vi "Control Panel No Objects.vi"(8 "error in (no error)":errorcluster) -> (0 "error out":errorcluster)   [LabVIEW 2009]
doc: "(Dynamic) A user-level application that simulates the physical front panel of the Instrument. Provide the user with buttons to manually control features of the instrument, and provide indicators of its current state."
uses:
  Math Operations/To Start and Stop (bare).vi
  Math Operations/To Center and Span (frequency).vi
  Function Generator.lvclass
  Tektronix AFG 3000 Series/Tektronix AFG 3000 Series.lvlib
  Tektronix AFG 3000 Series/controls.llb/Channel.ctl
  Math Operations/To Center and Span (bare).vi
  Math Operations/To Start and Stop (frequency).vi
  Tektronix AFG 3000 Series/controls.llb/Voltage.ctl
  Tektronix AFG 3000 Series/controls.llb/Frequency Mode.ctl
  Tektronix AFG 3000 Series/controls.llb/Sweep Frequency.ctl
  Tektronix AFG 3000 Series/controls.llb/Sweep Time Parameter.ctl
  Global/GPIB Numbers.vi
  Tektronix AFG 3000 Series/controls.llb/Waveform Shape.ctl
  Tektronix AFG 3000 Series/controls.llb/Sweep Spacing.ctl
panel:
  in  "Initial Cluster":T1
  in  "Ch2 on/off":bool
  in  "Ch1 on/off":bool
  out "Ready when blinking":bool
  in  "Set":bool
  in  "Read to control":bool
  in  "Read":bool
  in  "Copy actual to set":bool
  in  "Populate fields with member data":bool
  out "Start Freq.":dbl[unit]
  out "Stop Freq.":dbl[unit]
  out "Freq. Span":dbl[unit]
  out "Center Freq.":dbl[unit]
  out "Offset":dbl[unit]
  out "Amplitude":dbl[unit]
  out "High":dbl[unit]
  out "Low":dbl[unit]
  out "FM Source":u16(ring) items=["Internal", "External"]
  out "FM Modulation Waveform":u16(ring) items=["Sine", "Square", "Triangle", "Ramp", "Down Ramp", "Noise", "User 1", "User 2", "User 3", "User 4", "EMEMory", "EFILe"]
  out "FM Modulation Freq.":dbl[unit]=100.0
  out "FM Peak Deviation":dbl[unit]=100.0
  in  "FM Peak Deviation Set":dbl[unit]=100.0
  in  "FM Modulation Freq Set":dbl[unit]=100.0
  in  "FM Modulation Waveform Set":u16(ring) items=["Sine", "Square", "Triangle", "Ramp", "Down Ramp", "Noise", "User 1", "User 2", "User 3", "User 4", "EMEMory", "EFILe"]
  in  "FM Source Set":u16(ring) items=["Internal", "External"]
  out "AM Modulation Freq.":dbl[unit]=1000.0
  out "AM Modulation Waveform":u16(ring) items=["Sine", "Square", "Triangle", "Ramp", "Down Ramp", "Noise"]
  out "AM Source":u16(ring) items=["Internal", "External"]
  out "AM Modulation Depth":dbl
  in  "AM Modulation Depth Set":dbl
  in  "AM Modulation Freq. Set":dbl[unit]=1000.0
  in  "AM Modulation Waveform Set":u16(ring) items=["Sine", "Square", "Triangle", "Ramp", "Down Ramp", "Noise"]
  in  "AM Source Set":u16(ring) items=["Internal", "External"]
  out "Return Time":dbl[unit]
  out "Hold Time":dbl[unit]
  out "Sweep Time":dbl[unit]
  in  "Return Time Set":dbl[unit]
  in  "Hold Time Set":dbl[unit]
  in  "Sweep Time Set":dbl[unit] caption="Sweep time"
  out "Sweep Spacing":T2 items=["linear", "log"]
  in  "Sweep Spacing Set":T2 items=["linear", "log"]
  in  "Stop Freq. Set":dbl[unit]
  in  "Start Freq. Set":dbl[unit]
  out "Burst Mode":u16(ring)=1 items=["Triggered", "Gated"]
  out "Burst Count":i32=5
  in  "Burst Count Set":i32=5
  in  "Burst Mode Set":u16(ring)=1 items=["Triggered", "Gated"]
  out "Run Mode":u16(ring) items=["Continuous", "AM", "FM", "PM", "FSK", "PWM", "Sweep", "Burst"]
  in  "Run Mode Set":u16(ring) items=["Continuous", "AM", "FM", "PM", "FSK", "PWM", "Sweep", "Burst"]
  out "Trailing Edge Time":dbl[unit]
  out "Leading Edge Time":dbl[unit]
  out "Duty Cycle (%)":dbl
  in  "Duty Cycle Set (%)":dbl=50.0
  in  "Trailing Edge Time Set":dbl[unit]=5e-09 format="%#.6g"
  in  "Leading Edge Time Set":dbl[unit]=5e-09 format="%#.6g"
  out "Ramp Symm. (%)":dbl
  in  "Ramp Symm. Set (%)":dbl=50.0 min=0.0 max=100.0 step=1.0 format="%.2f"
  in  "Freq. Span Set":dbl[unit]
  in  "Center Freq. Set":dbl[unit]
  in  "Low Set":dbl[unit]
  in  "High Set":dbl[unit]
  in  "Amplitude Set":dbl[unit]
  in  "Offset Set":dbl[unit]
  in  "Exit":bool
  out "Waveform Shape":T3 items=["Sinusoid", "Square", "Pulse", "Ramp", "PRNoise", "DC", "SINC", "Gaussian", "Lorentz", "ERise", "EDecay", "Haversine", "User 1", "User 2", "User 3", "User 4", "EMemory", "EFile"]
  in  "Waveform Shape Set":T3 items=["Sinusoid", "Square", "Pulse", "Ramp", "PRNoise", "DC", "SINC", "Gaussian", "Lorentz", "ERise", "EDecay", "Haversine", "User 1", "User 2", "User 3", "User 4", "EMemory", "EFile"]
  out "Phase":dbl[unit]
  in  "Phase Set":dbl[unit]
  out "Frequency":dbl[unit]
  in  "Frequency Set":dbl[unit]
  in  "Channel":T4 items=["Channel 1", "Channel 2"]
  # "Tektronix AFG252 Function Generator Control Panel"
  # "VOLTAGE SETTINGS"
  # "SWEEP MODE SETTINGS"
  # "AM SETTINGS"
  # "GENERAL SETTINGS"
  # "RAMP SETTINGS"
  # "FM SETTINGS"
  # "Note: the program only sets\nthe values that are appropriate\nfor the run mode you select. I.e.,\nit won't set the FM settings if you\nselect \"Burst Mode\" here."
  # "PULSE SETTINGS"
  # "BURST MODE SETTINGS"
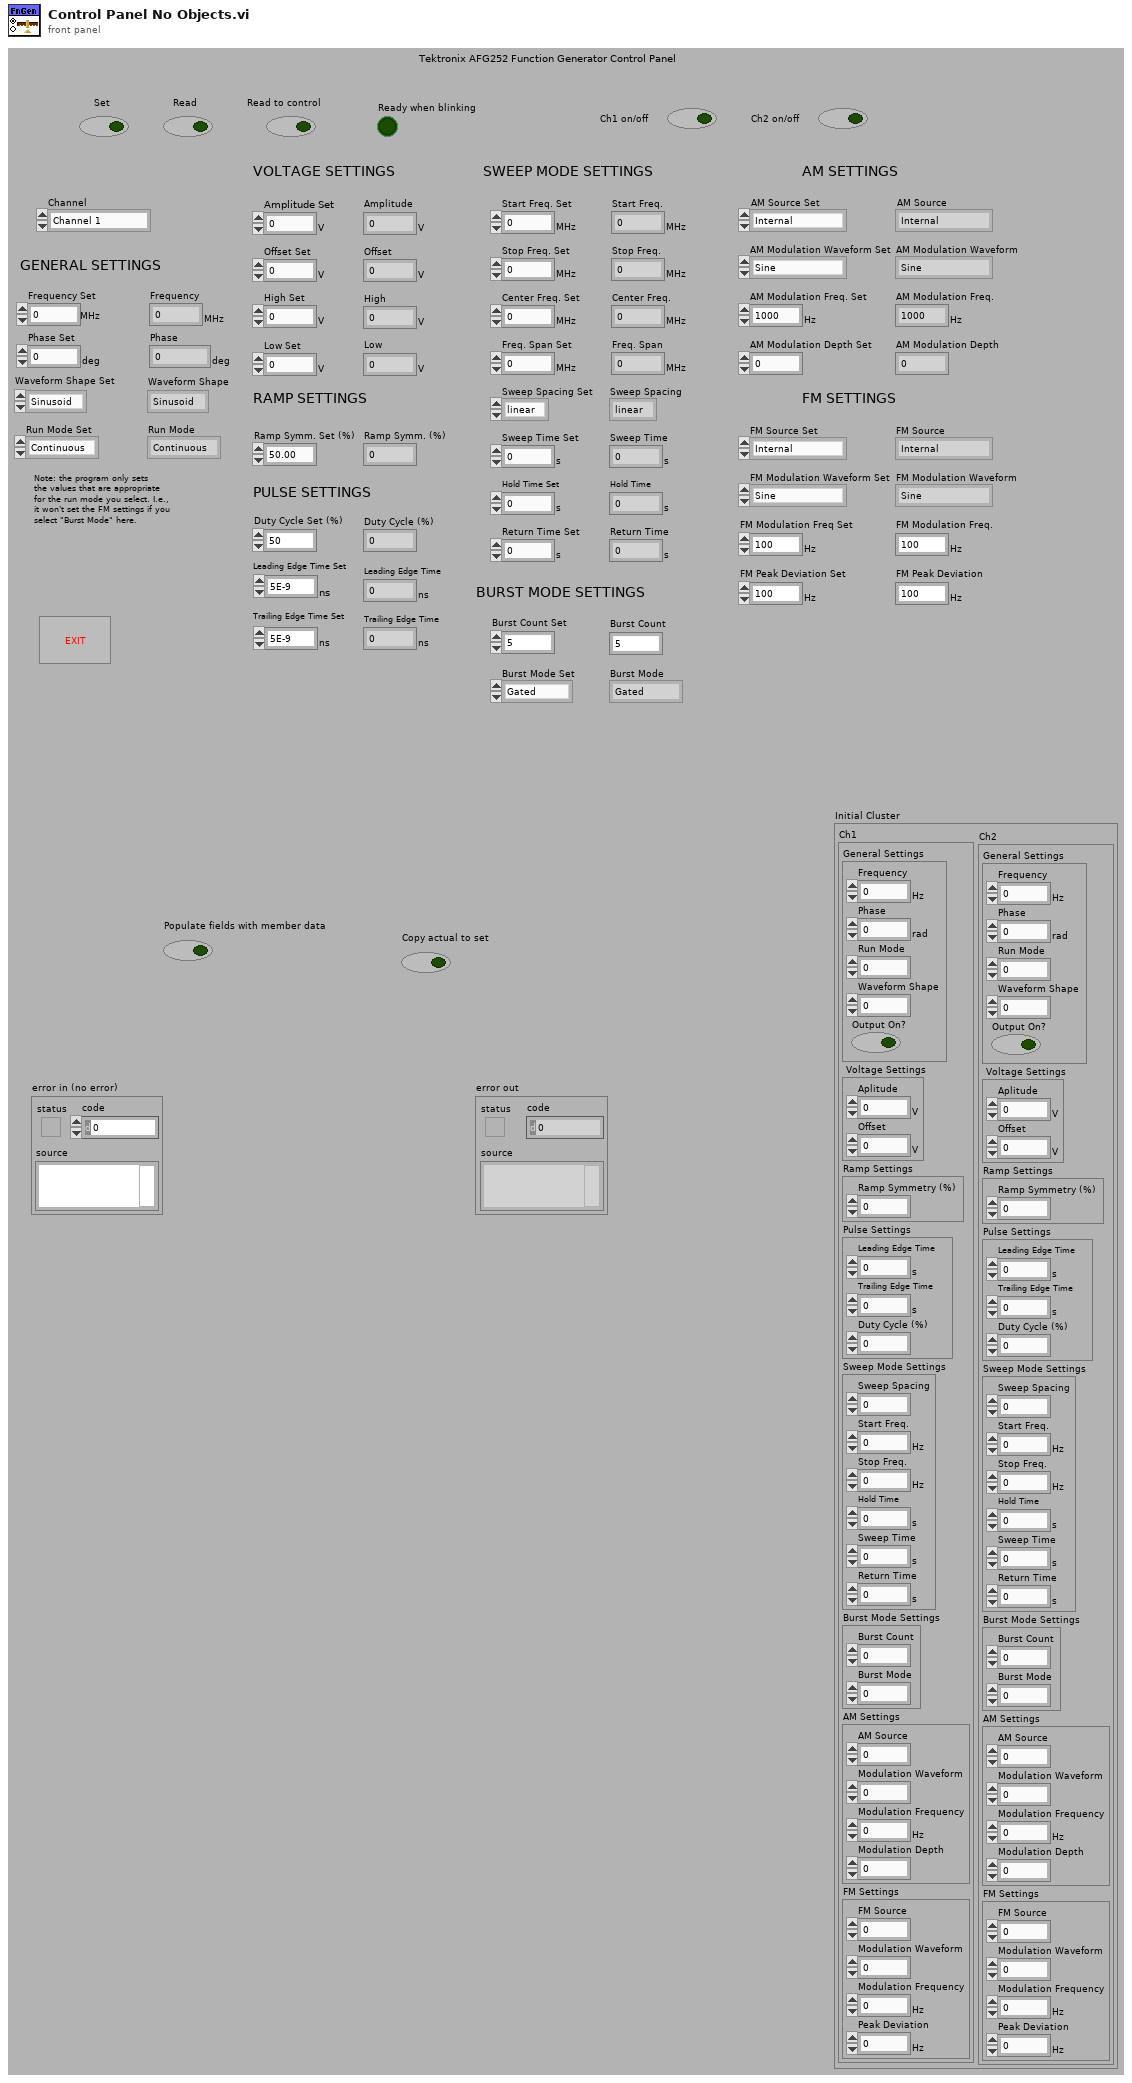
[diagram p1: front panel]
types:
  T1 = cluster{"Ch1":cluster{"General Settings":cluster{"Frequency":dbl[unit], "Phase":dbl[unit], "Run Mode":u16, "Waveform Shape":u16, "Output On?":bool}, " Voltage Settings":cluster{"Aplitude":dbl[unit], "Offset":dbl[unit]}, "Ramp Settings":cluster{"Ramp Symmetry (%)":dbl}, "Pulse Settings":cluster{"Leading Edge Time":dbl[unit], "Trailing Edge Time":dbl[unit], "Duty Cycle (%)":dbl}, "Sweep Mode Settings":cluster{"Sweep Spacing":u16, "Start Freq.":dbl[unit], "Stop Freq.":dbl[unit], "Hold Time":dbl[unit], "Sweep Time":dbl[unit], "Return Time":dbl[unit]}, "Burst Mode Settings":cluster{"Burst Count":i32, "Burst Mode":u16}, "AM Settings":cluster{"AM Source":u16, "Modulation Waveform":u16, "Modulation Frequency":dbl[unit], "Modulation Depth":dbl}, "FM Settings":cluster{"FM Source":u16, "Modulation Waveform":u16, "Modulation Frequency":dbl[unit], "Peak Deviation":dbl[unit]}}, "Ch2":cluster{"General Settings":cluster{"Frequency":dbl[unit], "Phase":dbl[unit], "Run Mode":u16, "Waveform Shape":u16, "Output On?":bool}, " Voltage Settings":cluster{"Aplitude":dbl[unit], "Offset":dbl[unit]}, "Ramp Settings":cluster{"Ramp Symmetry (%)":dbl}, "Pulse Settings":cluster{"Leading Edge Time":dbl[unit], "Trailing Edge Time":dbl[unit], "Duty Cycle (%)":dbl}, "Sweep Mode Settings":cluster{"Sweep Spacing":u16, "Start Freq.":dbl[unit], "Stop Freq.":dbl[unit], "Hold Time":dbl[unit], "Sweep Time":dbl[unit], "Return Time":dbl[unit]}, "Burst Mode Settings":cluster{"Burst Count":i32, "Burst Mode":u16}, "AM Settings":cluster{"AM Source":u16, "Modulation Waveform":u16, "Modulation Frequency":dbl[unit], "Modulation Depth":dbl}, "FM Settings":cluster{"FM Source":u16, "Modulation Waveform":u16, "Modulation Frequency":dbl[unit], "Peak Deviation":dbl[unit]}}}
  T2 = typedef "Sweep Spacing.ctl" = u16
  T3 = typedef "Waveform Shape.ctl" = u16
  T4 = typedef "Channel.ctl" = u16
  T5 = typedef "Voltage.ctl" = enum16{"amplitude", "offset", "high", "low", "high limit", "low limit"}
  T6 = typedef "Frequency Mode.ctl" = enum16{"CW", "Sweep"}
  T7 = typedef "Sweep Time Parameter.ctl" = enum16{"sweep time", "hold time", "return time"}
  T8 = typedef "Sweep Frequency.ctl" = enum16{"center", "span", "start", "stop"}
  T9 = cluster{"General Settings":cluster{"Frequency":dbl[unit], "Phase":dbl[unit], "Run Mode":u16, "Waveform Shape":u16, "Output On?":bool}, " Voltage Settings":cluster{"Aplitude":dbl[unit], "Offset":dbl[unit]}, "Ramp Settings":cluster{"Ramp Symmetry (%)":dbl}, "Pulse Settings":cluster{"Leading Edge Time":dbl[unit], "Trailing Edge Time":dbl[unit], "Duty Cycle (%)":dbl}, "Sweep Mode Settings":cluster{"Sweep Spacing":u16, "Start Freq.":dbl[unit], "Stop Freq.":dbl[unit], "Hold Time":dbl[unit], "Sweep Time":dbl[unit], "Return Time":dbl[unit]}, "Burst Mode Settings":cluster{"Burst Count":i32, "Burst Mode":u16}, "AM Settings":cluster{"AM Source":u16, "Modulation Waveform":u16, "Modulation Frequency":dbl[unit], "Modulation Depth":dbl}, "FM Settings":cluster{"FM Source":u16, "Modulation Waveform":u16, "Modulation Frequency":dbl[unit], "Peak Deviation":dbl[unit]}}
  T10 = cluster{"General Settings":cluster{"Frequency":dbl[unit], "Phase":dbl[unit], "Run Mode":u16, "Waveform Shape":u16, "Output On?":bool}, " Voltage Settings":cluster{"Aplitude":dbl[unit], "Offset":dbl[unit]}, "Ramp Settings":cluster{"Ramp Symmetry (%)":dbl}, "Pulse Settings":cluster{"Leading Edge Time":dbl[unit], "Trailing Edge Time":dbl[unit], "Duty Cycle (%)":dbl}, "Sweep Mode Settings":cluster{"Sweep Spacing":u16, "Start Freq.":dbl[unit], "Stop Freq.":dbl[unit], "Hold Time":dbl[unit], "Sweep Time":dbl[unit], "Return Time":dbl[unit]}, "Burst Mode Settings":cluster{"Burst Count":i32, "Burst Mode":u16}, "AM Settings":cluster{"AM Source":u16, "Modulation Waveform":u16, "Modulation Frequency":dbl[unit], "Modulation Depth":dbl}, "FM Settings":cluster{"FM Source":u16, "Modulation Waveform":u16, "Modulation Frequency":dbl[unit], "Peak Deviation":dbl[unit]}}[]
  T11 = typedef "GPIB Type Def.ctl" = cluster{"Name":string, "bus":dbl, "GPIB":dbl, "GPIB as string":string, "byte":i32, "VISA Resource Name":refnum<visa-resource-name>}
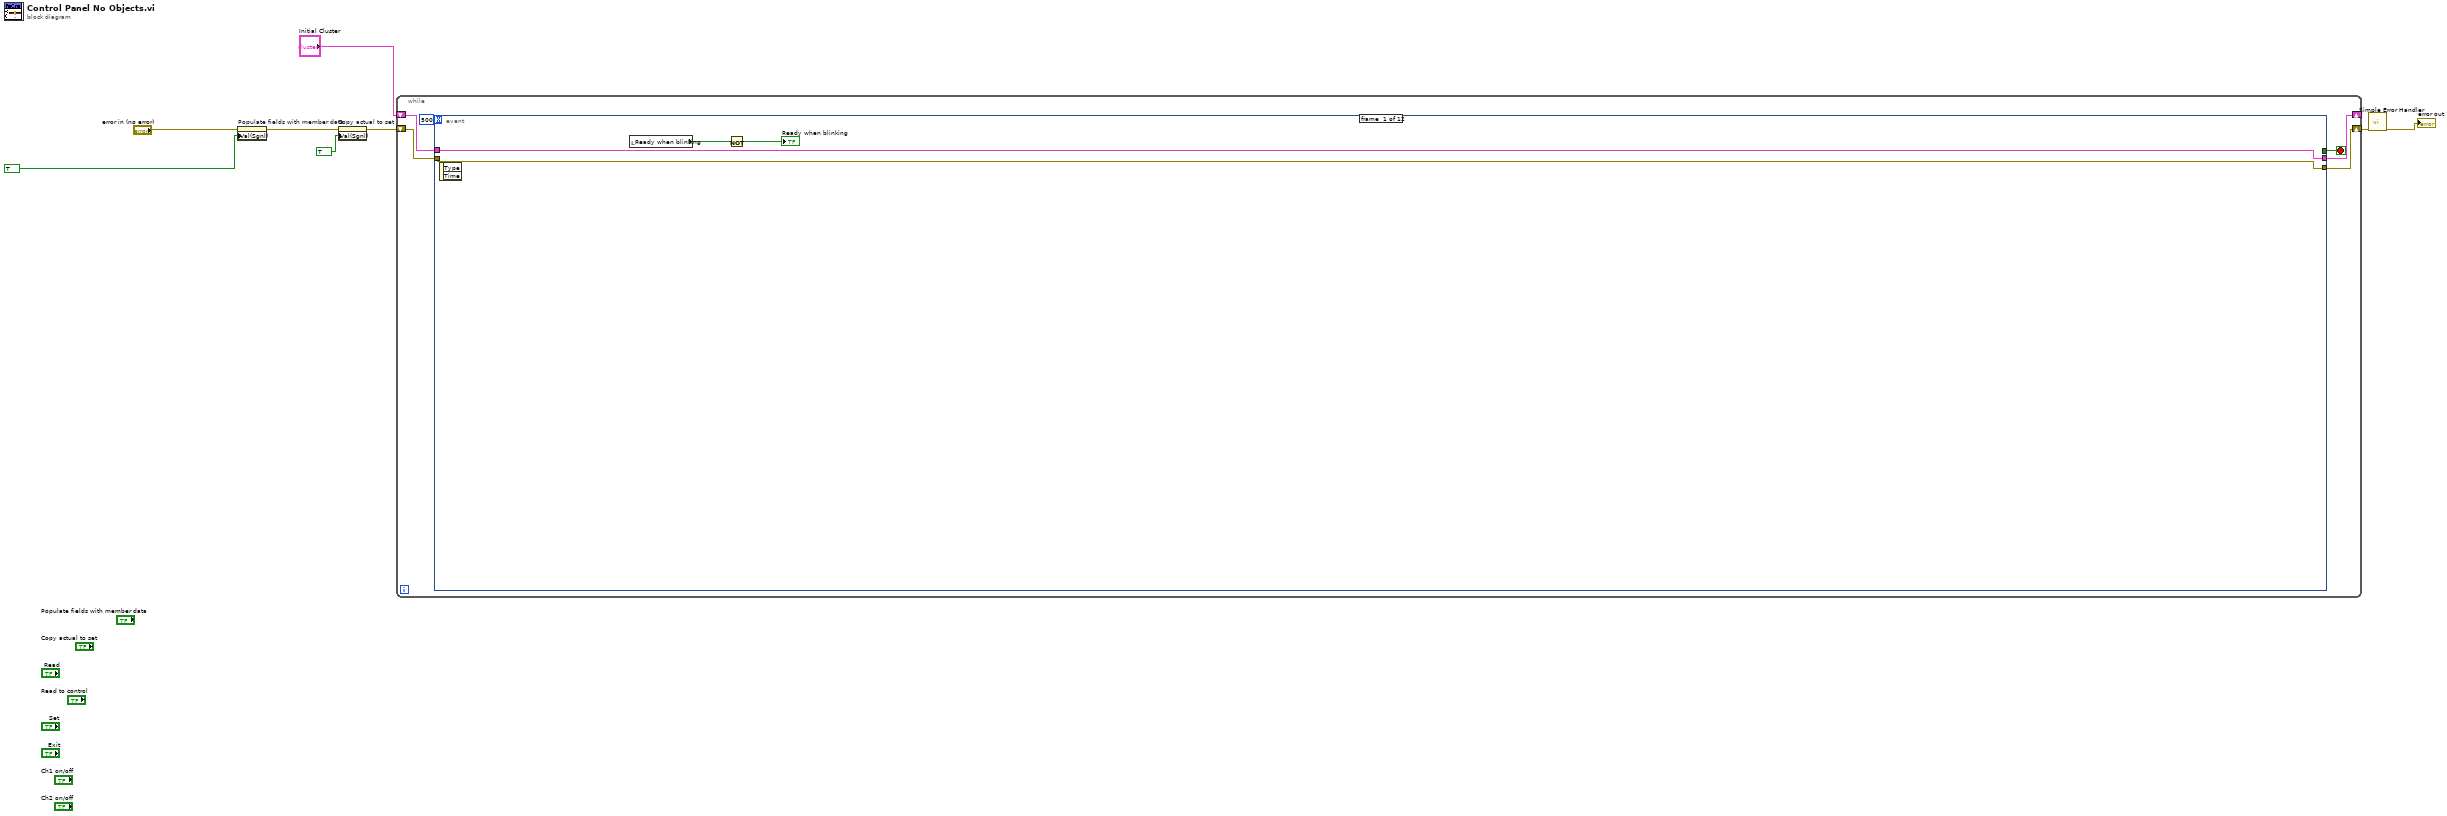
[diagram p0: block diagram]
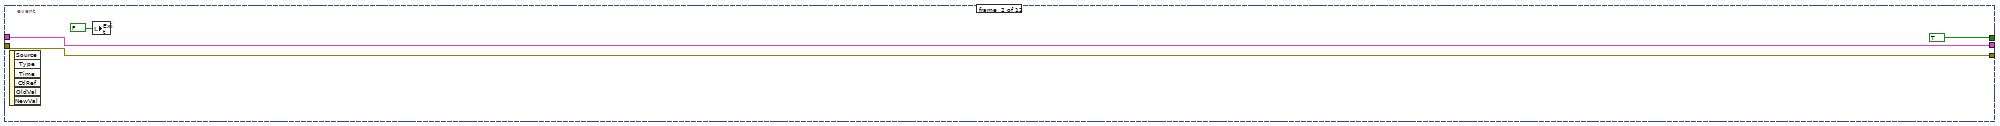
[diagram p2: hidden frame]
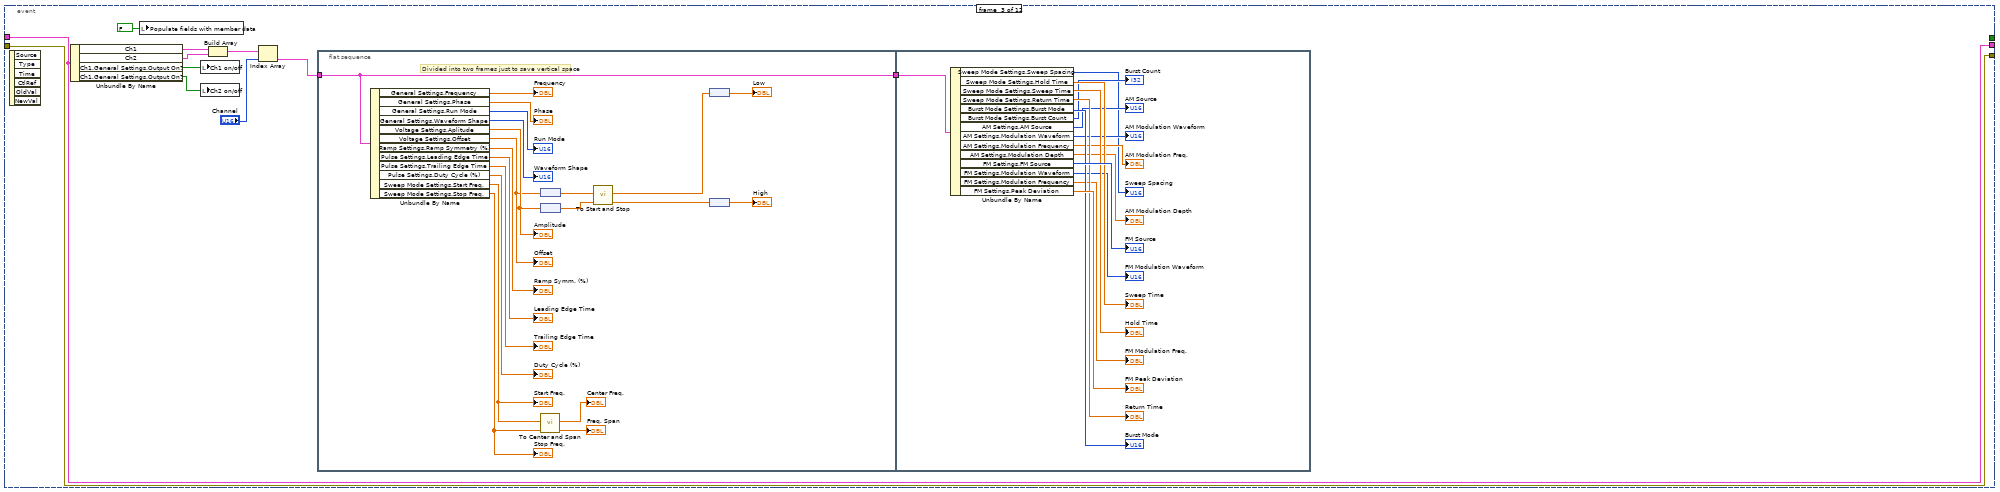
[diagram p3: hidden frame]
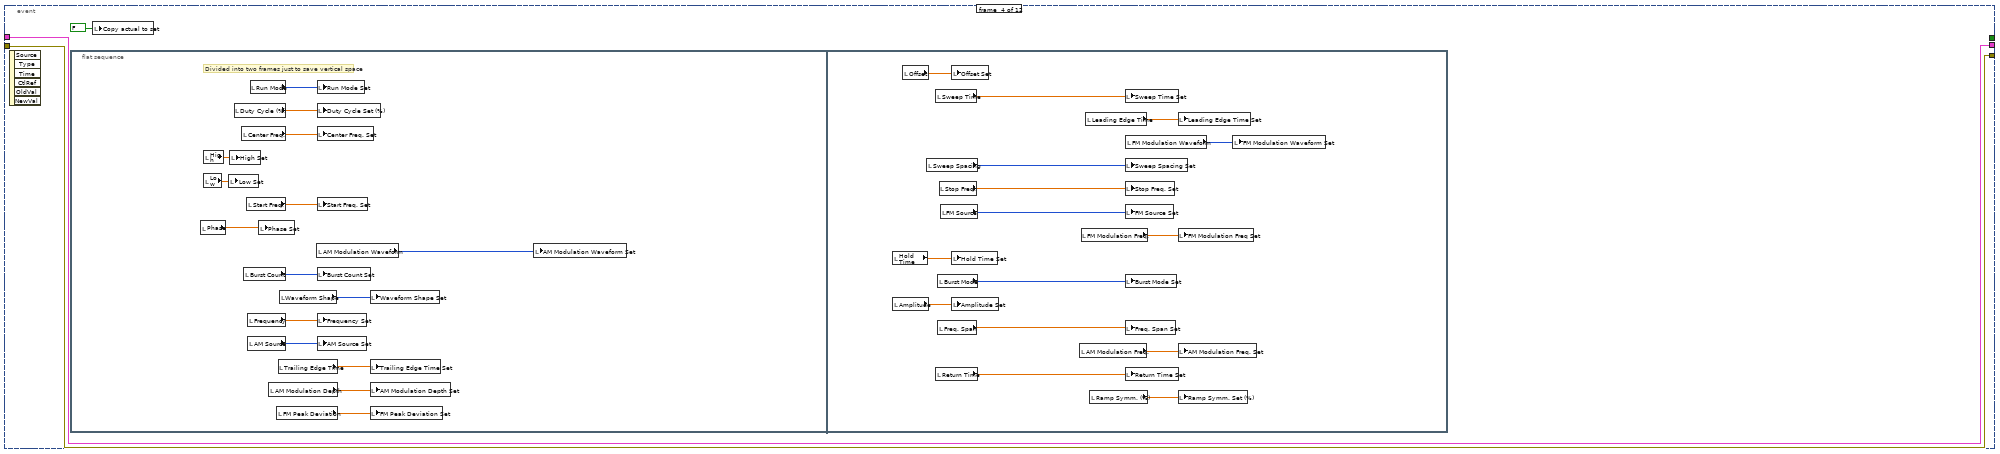
[diagram p4: hidden frame]
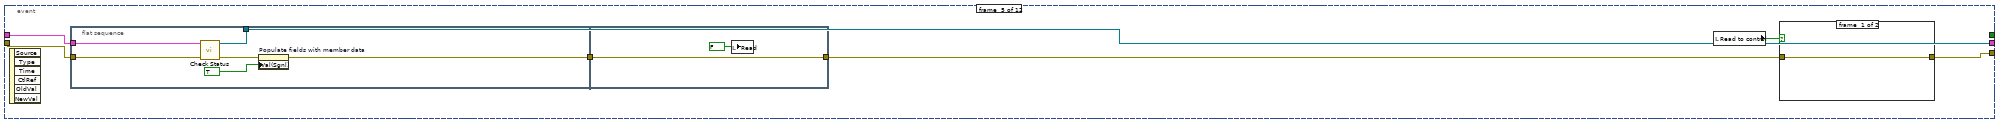
[diagram p5: hidden frame]
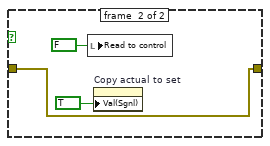
[diagram p6: hidden frame]
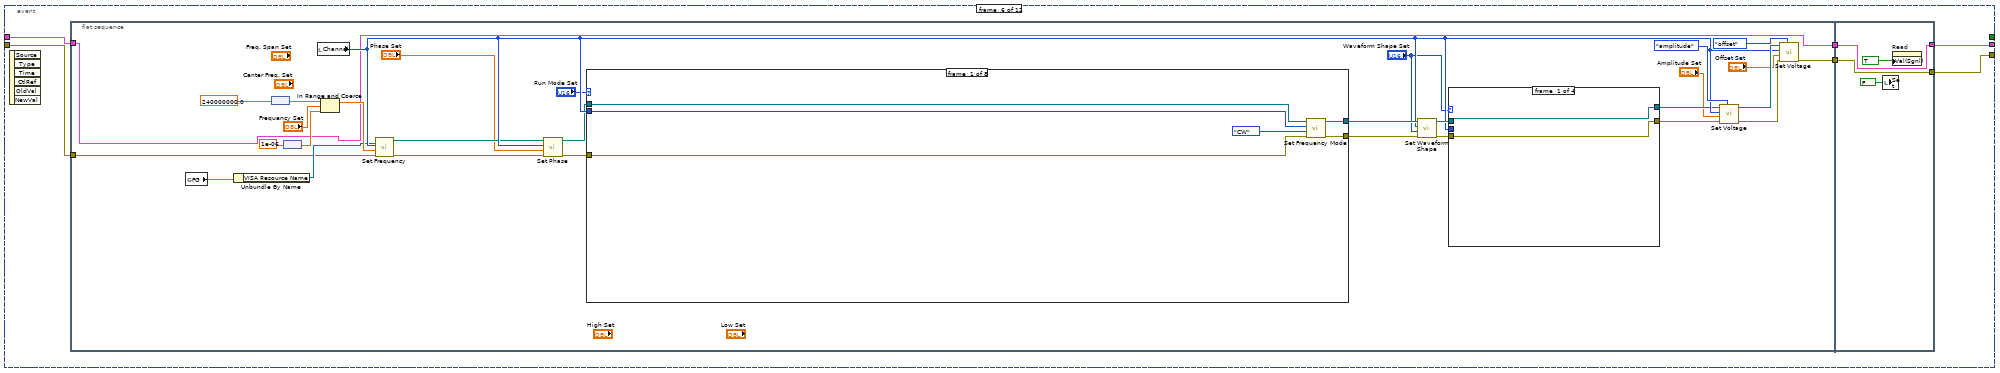
[diagram p7: hidden frame]
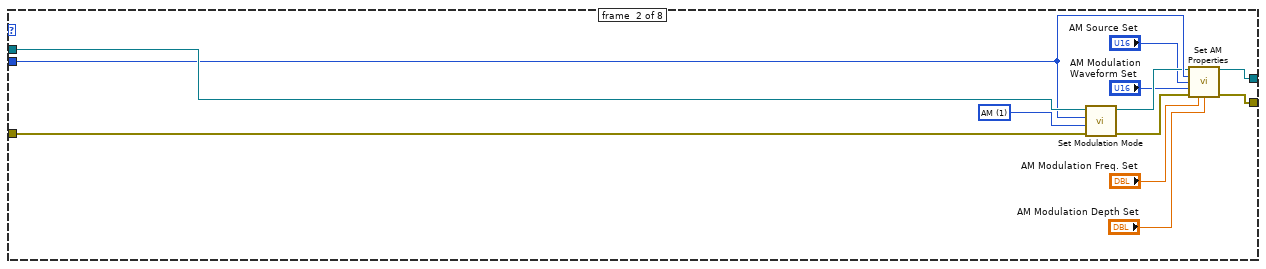
[diagram p8: hidden frame]
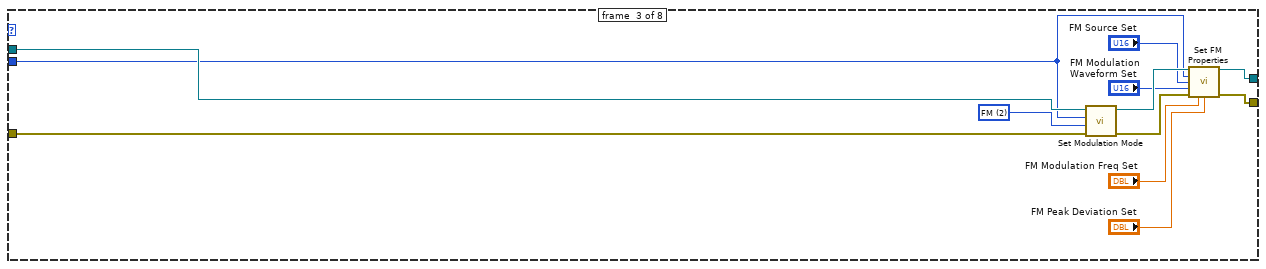
[diagram p9: hidden frame]
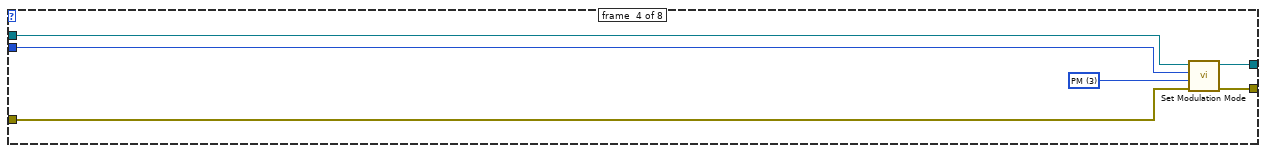
[diagram p10: hidden frame]
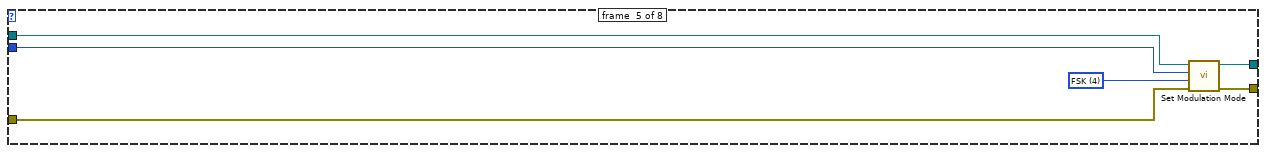
[diagram p11: hidden frame]
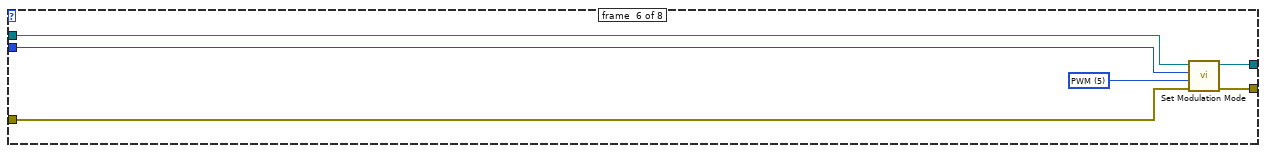
[diagram p12: hidden frame]
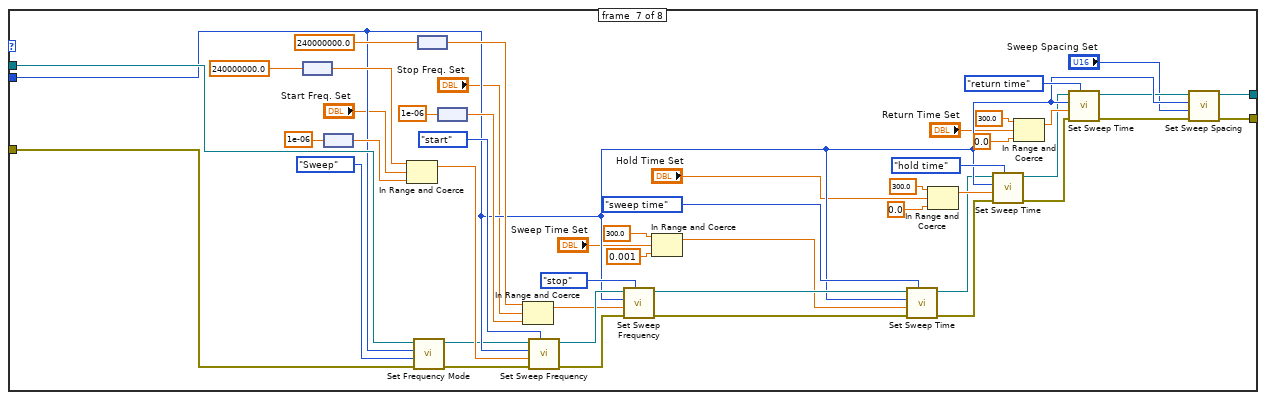
[diagram p13: hidden frame]
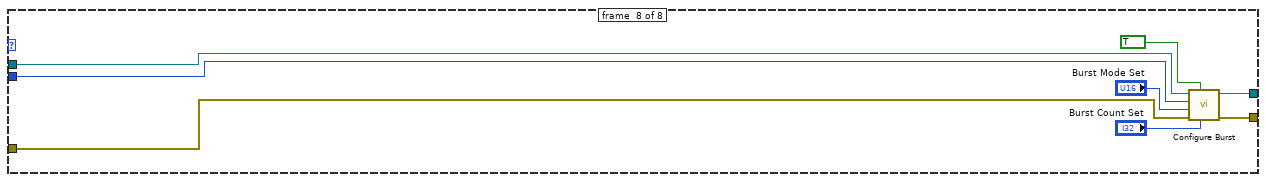
[diagram p14: hidden frame]
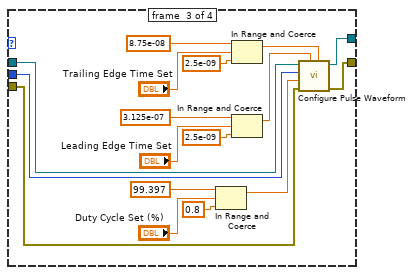
[diagram p16: hidden frame]
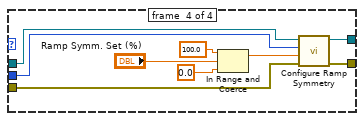
[diagram p17: hidden frame]
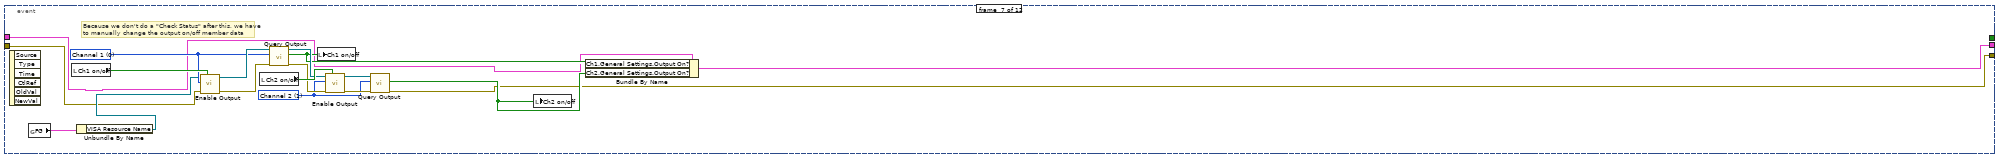
[diagram p18: hidden frame]
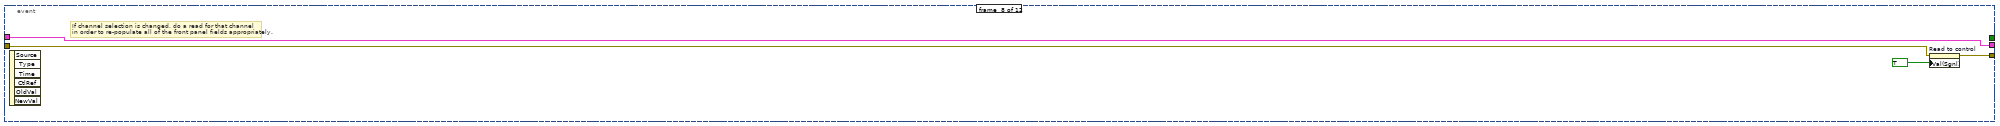
[diagram p19: hidden frame]
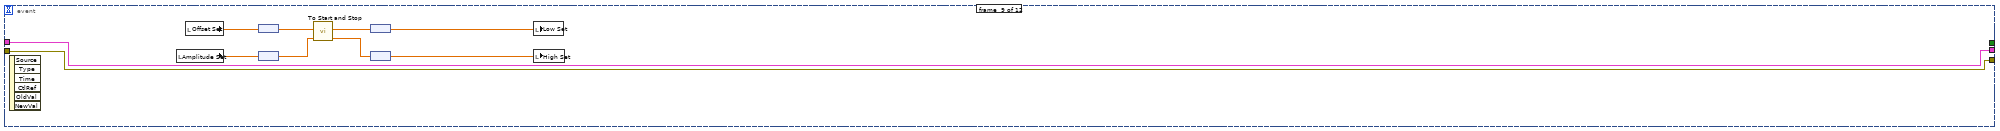
[diagram p20: hidden frame]
diagram:
  n1 = property on="Populate fields with member data" class="Bool (strict)"(error in="error in (no error)", "Val(Sgnl)"=TRUE ("Value (Signaling)")) -> (error out=w6:errorcluster)  [unwired: 1 in, 1 out]
  n2 = property on="Copy actual to set" class="Bool (strict)"(error in=w6, "Val(Sgnl)"=TRUE ("Value (Signaling)")) -> (error out=w5:errorcluster)  [unwired: 1 in, 1 out]
  n3 = while {
    shift-right: [w14] -> w4
    shift-left: w5 -> [w13]
    shift-right: [w11] -> _
    shift-left: "Initial Cluster" -> [w12]
    stop <- w9 stop-if-true
    n4 = event shown="[5] \"Set\": Value Change" {
      selector: _ -> [_ _ _ _ _ _ _ _ _ _ _ _]
      dyn-events: _ -> [_ _ _ _ _ _ _ _ _ _ _ _]
      timeout: 500 -> [_ _ _ _ _ _ _ _ _ _ _ _]
      tunnel: [w18 w19 w32 w71 w105 w124 w297 w316 w327 w337 w343 w349] -> w14
      tunnel: w13 -> [w18 w19 w32 w71 w106 w125 w299 w317 w327 w337 w343 w349]
      tunnel: [w17 w20 w31 w72 w103 w126 w304 w318 w328 w338 w344 w350] -> w11
      tunnel: w12 -> [w17 w20 w31 w72 w104 w127 w298 w318 w328 w338 w344 w350]
      tunnel: [_ TRUE ("Exit") _ _ _ _ _ _ _ _ _ _] -> w9
      event #0 {
        n5 = event-data() -> ()  [unwired: 3 out]
        n6 = local read "Ready when blinking"() -> (w16:bool)
        n7 = Not(x=w16) -> (.not. x?=→"Ready when blinking":bool)
      }
      event #1 {
        n8 = event-data() -> ()  [unwired: 7 out]
        n9 = local write "Exit"(FALSE ("Exit")) -> ()
      }
      event #2 {
        n10 = event-data() -> ()  [unwired: 7 out]
        n11 = Unbundle By Name(w31) -> ("Ch1"=w29:T9, "Ch2"=w30:T9, "Ch1.General Settings.Output On?"=w26:bool, "Ch1.General Settings.Output On?"=w25:bool)
        n12 = local write "Populate fields with member data"(FALSE ("Populate fields with member data")) -> ()
        n13 = local write "Ch1 on/off"(w26) -> ()
        n14 = local write "Ch2 on/off"(w25) -> ()
        n15 = Build Array(w29, w30) -> (w28:T10)
        n16 = Index Array(array=w28, index="Channel") -> (element=w24:T9)
        n17 = flat-sequence {
          tunnel: w24 -> [w34]
          tunnel: [w34] -> w23
          tunnel: w23 -> [w55]
          frame #0 {
            # "Divided into two frames just to save vertical space"
            n18 = Unbundle By Name(w34) -> ("General Settings.Frequency"=→"Frequency":dbl[unit], "General Settings.Phase"=→"Phase":dbl[unit], "General Settings.Run Mode"=→"Run Mode":u16, "General Settings.Waveform Shape"=→"Waveform Shape":u16, "Voltage Settings.Aplitude"=w42:dbl[unit], "Voltage Settings.Offset"=w41:dbl[unit], "Ramp Settings.Ramp Symmetry (%)"=→"Ramp Symm. (%)":dbl, "Pulse Settings.Leading Edge Time"=→"Leading Edge Time":dbl[unit], "Pulse Settings.Trailing Edge Time"=→"Trailing Edge Time":dbl[unit], "Pulse Settings.Duty Cycle (%)"=→"Duty Cycle (%)":dbl, "Sweep Mode Settings.Start Freq."=w36:dbl[unit], "Sweep Mode Settings.Stop Freq."=w35:dbl[unit])
            "Amplitude" <- w42
            "Offset" <- w41
            "Stop Freq." <- w35
            "Start Freq." <- w36
            n19 = node(w41) -> (w51:dbl)
            n20 = node(w42) -> (w52:dbl)
            n21 = call-poly "To Center and Span.vi"("stop"=w35, "start"=w36) -> ("span"=→"Freq. Span":dbl[unit], "center"=→"Center Freq.":dbl[unit])  [unwired: 4 out]
            n22 = call-poly "To Start and Stop.vi"("span"=w52, "center"=w51) -> ("stop"=w49:dbl, "start"=w50:dbl)  [unwired: 4 out]
            n23 = node(w50) -> (→"Low":dbl[unit])
            n24 = node(w49) -> (→"High":dbl[unit])
          }
          frame #1 {
            n25 = Unbundle By Name(w55) -> ("Sweep Mode Settings.Sweep Spacing"=→"Sweep Spacing":u16, "Sweep Mode Settings.Hold Time"=→"Sweep Time":dbl[unit], "Sweep Mode Settings.Sweep Time"=→"Hold Time":dbl[unit], "Sweep Mode Settings.Return Time"=→"Return Time":dbl[unit], "Burst Mode Settings.Burst Mode"=→"Burst Mode":u16, "Burst Mode Settings.Burst Count"=→"Burst Count":i32, "AM Settings.AM Source"=→"AM Source":u16, "AM Settings.Modulation Waveform"=→"AM Modulation Waveform":u16, "AM Settings.Modulation Frequency"=→"AM Modulation Freq.":dbl[unit], "AM Settings.Modulation Depth"=→"AM Modulation Depth":dbl, "FM Settings.FM Source"=→"FM Source":u16, "FM Settings.Modulation Waveform"=→"FM Modulation Waveform":u16, "FM Settings.Modulation Frequency"=→"FM Modulation Freq.":dbl[unit], "FM Settings.Peak Deviation"=→"FM Peak Deviation":dbl[unit])
          }
        }
      }
      event #3 {
        n26 = event-data() -> ()  [unwired: 7 out]
        n27 = flat-sequence {
          frame #0 {
            # "Divided into two frames just to save vertical space"
            n28 = local read "Phase"() -> (w84:dbl[unit])
            n29 = local read "High"() -> (w83:dbl[unit])
            n30 = local read "Low"() -> (w82:dbl[unit])
            n31 = local write "Low Set"(w82) -> ()
            n32 = local write "High Set"(w83) -> ()
            n33 = local read "Duty Cycle (%)"() -> (w81:dbl)
            n34 = local read "Center Freq."() -> (w78:dbl[unit])
            n35 = local read "Burst Count"() -> (w77:i32)
            n36 = local read "Start Freq."() -> (w79:dbl[unit])
            n37 = local read "Frequency"() -> (w87:dbl[unit])
            n38 = local read "AM Source"() -> (w76:u16)
            n39 = local read "Run Mode"() -> (w85:u16)
            n40 = local write "Phase Set"(w84) -> ()
            n41 = local read "AM Modulation Depth"() -> (w74:dbl)
            n42 = local read "FM Peak Deviation"() -> (w73:dbl[unit])
            n43 = local read "Trailing Edge Time"() -> (w80:dbl[unit])
            n44 = local read "Waveform Shape"() -> (w86:T3)
            n45 = local read "AM Modulation Waveform"() -> (w75:u16)
            n46 = local write "Run Mode Set"(w85) -> ()
            n47 = local write "Duty Cycle Set (%)"(w81) -> ()
            n48 = local write "Center Freq. Set"(w78) -> ()
            n49 = local write "Start Freq. Set"(w79) -> ()
            n50 = local write "Burst Count Set"(w77) -> ()
            n51 = local write "Frequency Set"(w87) -> ()
            n52 = local write "AM Source Set"(w76) -> ()
            n53 = local write "Waveform Shape Set"(w86) -> ()
            n54 = local write "Trailing Edge Time Set"(w80) -> ()
            n55 = local write "AM Modulation Depth Set"(w74) -> ()
            n56 = local write "FM Peak Deviation Set"(w73) -> ()
            n57 = local write "AM Modulation Waveform Set"(w75) -> ()
          }
          frame #1 {
            n58 = local read "Hold Time"() -> (w96:dbl[unit])
            n59 = local read "Amplitude"() -> (w88:dbl[unit])
            n60 = local read "Offset"() -> (w89:dbl[unit])
            n61 = local read "Sweep Spacing"() -> (w94:T2)
            n62 = local read "Sweep Time"() -> (w95:dbl[unit])
            n63 = local read "Return Time"() -> (w97:dbl[unit])
            n64 = local read "Burst Mode"() -> (w98:u16)
            n65 = local read "Freq. Span"() -> (w93:dbl[unit])
            n66 = local read "Stop Freq."() -> (w92:dbl[unit])
            n67 = local read "FM Source"() -> (w100:u16)
            n68 = local write "Offset Set"(w89) -> ()
            n69 = local write "Hold Time Set"(w96) -> ()
            n70 = local write "Amplitude Set"(w88) -> ()
            n71 = local read "AM Modulation Freq."() -> (w99:dbl[unit])
            n72 = local read "FM Modulation Freq."() -> (w102:dbl[unit])
            n73 = local read "Leading Edge Time"() -> (w91:dbl[unit])
            n74 = local read "Ramp Symm. (%)"() -> (w90:dbl)
            n75 = local write "Sweep Time Set"(w95) -> ()
            n76 = local write "Sweep Spacing Set"(w94) -> ()
            n77 = local write "Stop Freq. Set"(w92) -> ()
            n78 = local write "FM Source Set"(w100) -> ()
            n79 = local write "Burst Mode Set"(w98) -> ()
            n80 = local write "Freq. Span Set"(w93) -> ()
            n81 = local write "Return Time Set"(w97) -> ()
            n82 = local read "FM Modulation Waveform"() -> (w101:u16)
            n83 = local write "Leading Edge Time Set"(w91) -> ()
            n84 = local write "FM Modulation Freq Set"(w102) -> ()
            n85 = local write "AM Modulation Freq. Set"(w99) -> ()
            n86 = local write "Ramp Symm. Set (%)"(w90) -> ()
            n87 = local write "FM Modulation Waveform Set"(w101) -> ()
          }
        }
        n88 = local write "Copy actual to set"(FALSE ("Copy actual to set")) -> ()
      }
      event #4 {
        n89 = event-data() -> ()  [unwired: 7 out]
        n90 = flat-sequence {
          tunnel: [w114] -> w107
          tunnel: w106 -> [w116]
          tunnel: w104 -> [w119]
          tunnel: [w118] -> w103
          tunnel: [w121] -> w108
          tunnel: w107 -> [w121]
          frame #0 {
            n91 = call-dynamic "Check Status.vi"("error in (no error)"=w116, "Function Generator in"=w119) -> ("error out"=w115:errorcluster, "Function Generator out"=w118:refnum<class "Function Generator.lvclass">)  [unwired: 8 out]
            n92 = property on="Populate fields with member data" class="Bool (strict)"(error in=w115, "Val(Sgnl)"=TRUE ("Value (Signaling)")) -> (error out=w114:errorcluster)  [unwired: 1 in, 1 out]
          }
          frame #1 {
            n93 = local write "Read"(FALSE ("Read")) -> ()
          }
        }
        n94 = local read "Read to control"() -> (w109:bool)
        n95 = case shown="True" w109 {
          tunnel: [w110 w112] -> w105
          tunnel: w108 -> [w110 w112]
          frame #0 {
          }
          frame #1 {
            n96 = local write "Read to control"(FALSE ("Read")) -> ()
            n97 = property on="Copy actual to set" class="Bool (strict)"("Val(Sgnl)"=TRUE ("Value (Signaling)")) -> ()  [unwired: 2 in, 2 out]
          }
        }
      }
      event #5 {
        n98 = event-data() -> ()  [unwired: 7 out]
        n99 = flat-sequence {
          tunnel: w127 -> [w129]
          tunnel: w125 -> [w128]
          tunnel: [w130] -> w123
          tunnel: [w129] -> w122
          tunnel: [w295] -> w124
          tunnel: [w296] -> w126
          tunnel: w123 -> [w295]
          tunnel: w122 -> [w296]
          frame #0 {
            n100 = global read "GPIB Numbers.vi" "FG"() -> (w132:T11)
            n101 = Unbundle By Name(w132) -> ("VISA Resource Name"=w131:refnum<visa-resource-name>)
            n102 = node(240000000.0 ("upper limit")) -> (w155:dbl[unit])
            n103 = node(1e-06 ("lower limit")) -> (w156:dbl[unit])
            n104 = local read "Channel"() -> (w145:T4)
            n105 = In Range and Coerce(upper limit=w155, x="Frequency Set", lower limit=w156) -> (coerced(x)=w150:dbl[unit])  [unwired: 1 out]
            n106 = call "Set Frequency.vi"("error in (no error)"=w128, "frequency"=w150, "Channel (0: Channel 1)"=w145, "VISA resource name"=w131) -> ("error out"=w143:errorcluster, "VISA resource name out"=w144:refnum<visa-resource-name>)  [unwired: 6 out]
            n107 = call "Set Phase.vi"("error in (no error)"=w143, "phase"="Phase Set", "Channel (0: Channel 1)"=w145, "VISA resource name"=w144) -> ("error out"=w141:errorcluster, "VISA resource name out"=w142:refnum<visa-resource-name>)  [unwired: 1 in, 5 out]
            n108 = case shown="0, Default" "Run Mode Set" {
              tunnel: w142 -> [w163 w175 w188 w193 w199 w206 w254 w262]
              tunnel: w141 -> [w162 w174 w187 w192 w198 w205 w253 w261]
              tunnel: w145 -> [w161 w173 w183 w191 w197 w204 w224 w260]
              tunnel: [w160 w166 w178 w190 w196 w202 w216 w258] -> w147
              tunnel: [w159 w165 w177 w189 w195 w201 w215 w257] -> w146
              frame #0 {
                n109 = call "Set Frequency Mode.vi"("error in (no error)"=w162, "Mode (0: CW)"=Frequency_Mode."CW", "Channel (0: Channel 1)"=w161, "VISA resource name"=w163) -> ("error out"=w159:errorcluster, "VISA resource name out"=w160:refnum<visa-resource-name>)  [unwired: 6 out]
              }
              frame #1 {
                w176 = u16 1 items=["n/a", "AM", "FM", "PM", "FSK", "PWM"] ("Modulation Mode (def: AM)")
                n110 = call "Set Modulation Mode.vi"("error in (no error)"=w174, "Modulation Mode (def: AM)"=w176, "Channel (0: Channel 1)"=w173, "VISA resource name"=w175) -> ("error out"=w171:errorcluster, "VISA resource name out"=w172:refnum<visa-resource-name>)  [unwired: 6 out]
                n111 = call "Set AM Properties.vi"("VISA resource name"=w172, "Channel (0: Channel 1)"=w173, "AM Source (0: Internal)"="AM Source Set", "Modulation Waveform (0: Sine)"="AM Modulation Waveform Set", "error in (no error)"=w171, "Modulation Frequency (1000 Hz)"="AM Modulation Freq. Set", "Modulation Depth (0 %)"="AM Modulation Depth Set") -> ("VISA resource name out"=w166:refnum<visa-resource-name>, "error out"=w165:errorcluster)  [unwired: 7 out]
              }
              frame #2 {
                w186 = u16 2 items=["n/a", "AM", "FM", "PM", "FSK", "PWM"] ("Modulation Mode (def: AM)")
                n112 = call "Set Modulation Mode.vi"("error in (no error)"=w187, "Modulation Mode (def: AM)"=w186, "Channel (0: Channel 1)"=w183, "VISA resource name"=w188) -> ("error out"=w185:errorcluster, "VISA resource name out"=w184:refnum<visa-resource-name>)  [unwired: 6 out]
                n113 = call "Set FM Properties.vi"("VISA resource name"=w184, "Channel (0: Channel 1)"=w183, "FM Source (0: Internal)"="FM Source Set", "Modulation Waveform (0: Sine)"="FM Modulation Waveform Set", "error in (no error)"=w185, "Modulation Frequency (100.00 Hz)"="FM Modulation Freq Set", "Peak Deviation (100.00 Hz)"="FM Peak Deviation Set") -> ("VISA resource name out"=w178:refnum<visa-resource-name>, "error out"=w177:errorcluster)  [unwired: 7 out]
              }
              frame #3 {
                w194 = u16 3 items=["n/a", "AM", "FM", "PM", "FSK", "PWM"] ("Modulation Mode (def: AM)")
                n114 = call "Set Modulation Mode.vi"("error in (no error)"=w192, "Modulation Mode (def: AM)"=w194, "Channel (0: Channel 1)"=w191, "VISA resource name"=w193) -> ("error out"=w189:errorcluster, "VISA resource name out"=w190:refnum<visa-resource-name>)  [unwired: 6 out]
              }
              frame #4 {
                w200 = u16 4 items=["n/a", "AM", "FM", "PM", "FSK", "PWM"] ("Modulation Mode (def: AM)")
                n115 = call "Set Modulation Mode.vi"("error in (no error)"=w198, "Modulation Mode (def: AM)"=w200, "Channel (0: Channel 1)"=w197, "VISA resource name"=w199) -> ("error out"=w195:errorcluster, "VISA resource name out"=w196:refnum<visa-resource-name>)  [unwired: 6 out]
              }
              frame #5 {
                w203 = u16 5 items=["n/a", "AM", "FM", "PM", "FSK", "PWM"] ("Modulation Mode (def: AM)")
                n116 = call "Set Modulation Mode.vi"("error in (no error)"=w205, "Modulation Mode (def: AM)"=w203, "Channel (0: Channel 1)"=w204, "VISA resource name"=w206) -> ("error out"=w201:errorcluster, "VISA resource name out"=w202:refnum<visa-resource-name>)  [unwired: 6 out]
              }
              frame #6 {
                n117 = node(240000000.0 ("upper limit")) -> (w247:dbl[unit])
                n118 = node(1e-06 ("lower limit")) -> (w248:dbl[unit])
                n119 = In Range and Coerce(upper limit=w247, x="Start Freq. Set", lower limit=w248) -> (coerced(x)=w225:dbl[unit])  [unwired: 1 out]
                n120 = call "Set Frequency Mode.vi"("error in (no error)"=w253, "Mode (0: CW)"=Frequency_Mode."Sweep", "Channel (0: Channel 1)"=w224, "VISA resource name"=w254) -> ("error out"=w207:errorcluster, "VISA resource name out"=w208:refnum<visa-resource-name>)  [unwired: 6 out]
                n121 = node(240000000.0 ("upper limit")) -> (w244:dbl[unit])
                n122 = node(1e-06 ("lower limit")) -> (w245:dbl[unit])
                n123 = In Range and Coerce(upper limit=w244, x="Stop Freq. Set", lower limit=w245) -> (coerced(x)=w241:dbl[unit])  [unwired: 1 out]
                n124 = call "Set Sweep Frequency.vi"("Sweep Frequency"=Sweep_Frequency."start", "error in (no error)"=w207, "frequency"=w225, "Channel (0: Channel 1)"=w224, "VISA resource name"=w208) -> ("error out"=w242:errorcluster, "VISA resource name out"=w243:refnum<visa-resource-name>)  [unwired: 5 out]
                n125 = call "Set Sweep Frequency.vi"("Sweep Frequency"=Sweep_Frequency."stop", "error in (no error)"=w242, "frequency"=w241, "Channel (0: Channel 1)"=w224, "VISA resource name"=w243) -> ("error out"=w236:errorcluster, "VISA resource name out"=w237:refnum<visa-resource-name>)  [unwired: 5 out]
                n126 = In Range and Coerce(upper limit=dbl[unit] 300.0, x="Sweep Time Set", lower limit=dbl[unit] 0.001) -> (coerced(x)=w231:dbl[unit])  [unwired: 1 out]
                n127 = call "Set Sweep Time.vi"("Sweep Time Param (sweep time)"=Sweep_Time_Parameter."sweep time", "error in (no error)"=w236, "time"=w231, "Channel (0: Channel 1)"=w224, "VISA resource name"=w237) -> ("error out"=w221:errorcluster, "VISA resource name out"=w222:refnum<visa-resource-name>)  [unwired: 5 out]
                n128 = In Range and Coerce(upper limit=dbl[unit] 300.0, x="Hold Time Set", lower limit=dbl[unit] 0.0) -> (coerced(x)=w228:dbl[unit])  [unwired: 1 out]
                n129 = call "Set Sweep Time.vi"("Sweep Time Param (sweep time)"=Sweep_Time_Parameter."hold time", "error in (no error)"=w221, "time"=w228, "Channel (0: Channel 1)"=w224, "VISA resource name"=w222) -> ("error out"=w219:errorcluster, "VISA resource name out"=w220:refnum<visa-resource-name>)  [unwired: 5 out]
                n130 = In Range and Coerce(upper limit=dbl[unit] 300.0, x="Return Time Set", lower limit=dbl[unit] 0.0) -> (coerced(x)=w227:dbl[unit])  [unwired: 1 out]
                n131 = call "Set Sweep Time.vi"("Sweep Time Param (sweep time)"=Sweep_Time_Parameter."return time", "error in (no error)"=w219, "time"=w227, "Channel (0: Channel 1)"=w224, "VISA resource name"=w220) -> ("error out"=w217:errorcluster, "VISA resource name out"=w218:refnum<visa-resource-name>)  [unwired: 5 out]
                n132 = call "Set Sweep Spacing.vi"("error in (no error)"=w217, "Sweep spacing (linear)"="Sweep Spacing Set", "Channel (0: Channel 1)"=w224, "VISA resource name"=w218) -> ("error out"=w215:errorcluster, "VISA resource name out"=w216:refnum<visa-resource-name>)  [unwired: 6 out]
              }
              frame #7 {
                n133 = call "Configure Burst.vi"("Burst Count (5)"="Burst Count Set", "Enable Burst (T: Enable)"=TRUE, "error in (no error)"=w261, "Burst Mode (0: Triggered)"="Burst Mode Set", "Channel (0: Channel 1)"=w260, "VISA resource name"=w262) -> ("error out"=w257:errorcluster, "VISA resource name out"=w258:refnum<visa-resource-name>)  [unwired: 4 out]
              }
            }
            n134 = call "Set Waveform Shape.vi"("error in (no error)"=w146, "Waveform Shape"="Waveform Shape Set", "Channel (0: Channel 1)"=w145, "VISA resource name"=w147) -> ("error out"=w148:errorcluster, "VISA resource name out"=w149:refnum<visa-resource-name>)  [unwired: 6 out]
            n135 = case shown="0, Default" "Waveform Shape Set" {
              tunnel: w149 -> [w264 w266 w283 w292]
              tunnel: w148 -> [w263 w265 w282 w291]
              tunnel: [w264 w266 w268 w285] -> w138
              tunnel: [w263 w265 w267 w284] -> w137
              tunnel: w145 -> [_ _ w272 w287]
              frame #0 {
              }
              frame #1 {
              }
              frame #2 {
                n136 = In Range and Coerce(upper limit=99.397, x="Duty Cycle Set (%)", lower limit=0.8) -> (coerced(x)=w273:dbl)  [unwired: 1 out]
                n137 = In Range and Coerce(upper limit=dbl[unit] 8.75e-08, x="Trailing Edge Time Set", lower limit=dbl[unit] 2.5e-09) -> (coerced(x)=w276:dbl[unit])  [unwired: 1 out]
                n138 = In Range and Coerce(upper limit=dbl[unit] 3.125e-07, x="Leading Edge Time Set", lower limit=dbl[unit] 2.5e-09) -> (coerced(x)=w279:dbl[unit])  [unwired: 1 out]
                n139 = call "Configure Pulse Waveform.vi"("Trailing Edge Time (5.0E-9 s)"=w276, "Leading Edge Time (5.0E-9 s)"=w279, "error in (no error)"=w282, "Duty Cycle (50%)"=w273, "Channel (0: Channel 1)"=w272, "VISA resource name"=w283) -> ("error out"=w267:errorcluster, "VISA resource name out"=w268:refnum<visa-resource-name>)  [unwired: 1 in, 3 out]
              }
              frame #3 {
                n140 = In Range and Coerce(upper limit=100.0, x="Ramp Symm. Set (%)", lower limit=0.0) -> (coerced(x)=w288:dbl)  [unwired: 1 out]
                n141 = call "Configure Ramp Symmetry.vi"("error in (no error)"=w291, "Ramp Symmetry (50.00 %)"=w288, "Channel (0: Channel 1)"=w287, "VISA resource name"=w292) -> ("error out"=w284:errorcluster, "VISA resource name out"=w285:refnum<visa-resource-name>)  [unwired: 6 out]
              }
            }
            n142 = call "Set Voltage.vi"("Voltage Param (amplitude)"=Voltage."amplitude", "error in (no error)"=w137, "voltage"="Amplitude Set", "Channel (0: Channel 1)"=w145, "VISA resource name"=w138) -> ("error out"=w153:errorcluster, "VISA resource name out"=w152:refnum<visa-resource-name>)  [unwired: 5 out]
            n143 = call "Set Voltage.vi"("Voltage Param (amplitude)"=Voltage."offset", "error in (no error)"=w153, "voltage"="Offset Set", "Channel (0: Channel 1)"=w145, "VISA resource name"=w152) -> ("error out"=w130:errorcluster)  [unwired: 6 out]
          }
          frame #1 {
            n144 = local write "Set"(FALSE ("Set")) -> ()
            n145 = property on="Read" class="Bool (strict)"("Val(Sgnl)"=TRUE ("Value (Signaling)")) -> ()  [unwired: 2 in, 2 out]
          }
        }
      }
      event #6 {
        w305 = T4 1 items=["Channel 1", "Channel 2"] ("Channel (0: Channel 1)")
        w306 = T4 0 items=["Channel 1", "Channel 2"] ("Channel (0: Channel 1)")
        # "Because we don't do a \"Check Status\" after this, we have \nto manually change the output on/off member data"
        n146 = event-data() -> ()  [unwired: 7 out]
        n147 = global read "GPIB Numbers.vi" "FG"() -> (w301:T11)
        n148 = local read "Ch1 on/off"() -> (w314:bool)
        n149 = Unbundle By Name(w301) -> ("VISA Resource Name"=w300:refnum<visa-resource-name>)
        n150 = call "Enable Output.vi"("Enable Output (T: Enable)"=w314, "error in (no error)"=w299, "Channel (0: Channel 1)"=w306, "VISA resource name"=w300) -> ("error out"=w309:errorcluster, "VISA resource name out"=w312:refnum<visa-resource-name>)  [unwired: 6 out]
        n151 = local read "Ch2 on/off"() -> (w313:bool)
        n152 = call "Query Output.vi"("error in (no error)"=w309, "Channel (0: Channel 1)"=w306, "VISA resource name"=w312) -> ("error out"=w308:errorcluster, "Output Enabled?"=w303:bool, "VISA resource name out"=w311:refnum<visa-resource-name>)  [unwired: 6 out]
        n153 = local write "Ch1 on/off"(w303) -> ()
        n154 = call "Enable Output.vi"("Enable Output (T: Enable)"=w313, "error in (no error)"=w308, "Channel (0: Channel 1)"=w305, "VISA resource name"=w311) -> ("error out"=w307:errorcluster, "VISA resource name out"=w310:refnum<visa-resource-name>)  [unwired: 6 out]
        n155 = call "Query Output.vi"("error in (no error)"=w307, "Channel (0: Channel 1)"=w305, "VISA resource name"=w310) -> ("error out"=w297:errorcluster, "Output Enabled?"=w302:bool)  [unwired: 7 out]
        n156 = local write "Ch2 on/off"(w302) -> ()
        n157 = Bundle By Name(cluster=w298, "Ch1.General Settings.Output On?"=w303, "Ch2.General Settings.Output On?"=w302) -> (w304:T1)
      }
      event #7 {
        # "If channel selection is changed, do a read for that channel\nin order to re-populate all of the front panel fields appropriately."
        n158 = event-data() -> ()  [unwired: 7 out]
        n159 = property on="Read to control" class="Bool (strict)"(error in=w317, "Val(Sgnl)"=TRUE ("Value (Signaling)")) -> (error out=w316:errorcluster)  [unwired: 1 in, 1 out]
      }
      event #8 {
        n160 = event-data() -> ()  [unwired: 7 out]
        n161 = local read "Amplitude Set"() -> (w321:dbl[unit])
        n162 = local read "Offset Set"() -> (w322:dbl[unit])
        n163 = node(w322) -> (w324:dbl)
        n164 = node(w321) -> (w323:dbl)
        n165 = call-poly "To Start and Stop.vi"("span"=w323, "center"=w324) -> ("stop"=w326:dbl, "start"=w325:dbl)  [unwired: 4 out]
        n166 = node(w325) -> (w320:dbl[unit])
        n167 = node(w326) -> (w319:dbl[unit])
        n168 = local write "Low Set"(w320) -> ()
        n169 = local write "High Set"(w319) -> ()
      }
      event #9 {
        n170 = event-data() -> ()  [unwired: 7 out]
        n171 = local read "High Set"() -> (w332:dbl[unit])
        n172 = local read "Low Set"() -> (w331:dbl[unit])
        n173 = node(w331) -> (w336:dbl)
        n174 = node(w332) -> (w335:dbl)
        n175 = call-poly "To Center and Span.vi"("stop"=w335, "start"=w336) -> ("span"=w333:dbl, "center"=w334:dbl)  [unwired: 4 out]
        n176 = node(w334) -> (w330:dbl[unit])
        n177 = node(w333) -> (w329:dbl[unit])
        n178 = local write "Offset Set"(w330) -> ()
        n179 = local write "Amplitude Set"(w329) -> ()
      }
      event #10 {
        n180 = event-data() -> ()  [unwired: 7 out]
        n181 = local read "Start Freq. Set"() -> (w342:dbl[unit])
        n182 = local read "Stop Freq. Set"() -> (w341:dbl[unit])
        n183 = call-poly "To Center and Span.vi"("stop"=w341, "start"=w342) -> ("span"=w339:dbl[unit], "center"=w340:dbl[unit])  [unwired: 4 out]
        n184 = local write "Center Freq. Set"(w340) -> ()
        n185 = local write "Freq. Span Set"(w339) -> ()
      }
      event #11 {
        n186 = event-data() -> ()  [unwired: 7 out]
        n187 = local read "Center Freq. Set"() -> (w348:dbl[unit])
        n188 = local read "Freq. Span Set"() -> (w347:dbl[unit])
        n189 = call-poly "To Start and Stop.vi"("span"=w347, "center"=w348) -> ("stop"=w345:dbl[unit], "start"=w346:dbl[unit])  [unwired: 4 out]
        n190 = local write "Start Freq. Set"(w346) -> ()
        n191 = local write "Stop Freq. Set"(w345) -> ()
      }
    }
  }
  n192 = call <vilib>:"Simple Error Handler.vi"("error in (no error)"=w4) -> ("error out"=→"error out":errorcluster)  [unwired: 1 in, 7 out]
